vi "HAMEG_HMP2020.vi"() -> ()   [LabVIEW 2011, in "run.lvlib"]
uses:
  run.lvlib
panel:
  out "Boolean array":bool[](array[boolean])
  in  "Time":dbl[](array[numeric])=[0.1, 0.1]
  in  "Voltage":dbl[](array[numeric])=[0.5, 0.4] format="%.3f"
  in  "Current":dbl[](array[numeric])=[2.0, 2.0] format="%.3f"
  in  "Channel (Channel 1)":i32(ring)=1 items=["Channel 1"=1, "Channel 2"=2, "Channel 3"=3, "Channel 4"=4]
  in  "VISA resource name":refnum<visa-resource-name>="COM3"
  in  "stop":bool
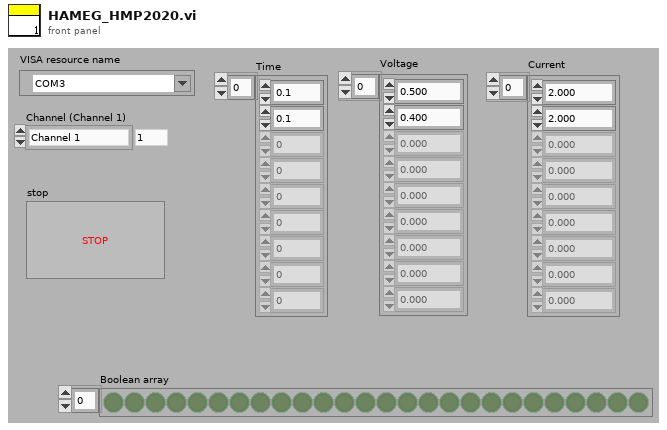
[diagram p1: front panel]
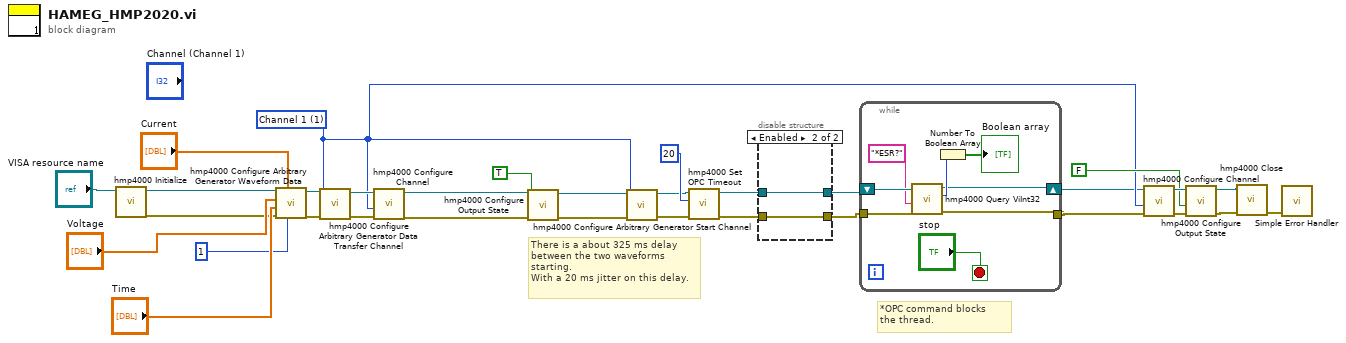
[diagram p0: block diagram]
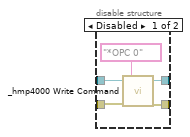
[diagram p2: hidden frame]
diagram:
  w3 = 1 items=["Channel 1"=1, "Channel 2"=2, "Channel 3"=3, "Channel 4"=4] ("Channel (Channel 1)")
  # "*OPC command blocks \nthe thread."
  # "There is a about 325 ms delay\nbetween the two waveforms \nstarting.\nWith a 20 ms jitter on this delay."
  n1 = call <instrlib>:"hmp4000 Initialize.vi"("VISA resource name"="VISA resource name") -> ("error out"=w4:errorcluster, "VISA resource name out"=w5:refnum<visa-resource-name>)  [unwired: 9 in]
  n2 = call <instrlib>:"hmp4000 Configure Arbitrary Generator Waveform Data.vi"("Repetition (0)"=1, "Current"="Current", "error in (no error)"=w4, "Time"="Time", "Voltage"="Voltage", "VISA resource name"=w5) -> ("error out"=w25:errorcluster, "VISA resource name out"=w26:refnum<visa-resource-name>)  [unwired: 4 in]
  n3 = call <instrlib>:"hmp4000 Configure Arbitrary Generator Data Transfer Channel.vi"("error in (no error)"=w25, "Channel (Channel 1)"=w3, "VISA resource name"=w26) -> ("error out"=w24:errorcluster, "VISA resource name out"=w23:refnum<visa-resource-name>)  [unwired: 7 in]
  n4 = call <instrlib>:"hmp4000 Configure Channel.vi"("error in (no error)"=w24, "Channel (Channel 1)"=w3, "VISA resource name"=w23) -> ("error out"=w6:errorcluster, "VISA resource name out"=w7:refnum<visa-resource-name>)  [unwired: 7 in]
  n5 = call <instrlib>:"hmp4000 Configure Output State.vi"("error in (no error)"=w6, "Output State (Off)"=TRUE, "VISA resource name"=w7) -> ("error out"=w8:errorcluster, "VISA resource name out"=w9:refnum<visa-resource-name>)  [unwired: 7 in]
  n6 = call <instrlib>:"hmp4000 Configure Arbitrary Generator Start Channel.vi"("error in (no error)"=w8, "Channel (Channel 1)"=w3, "VISA resource name"=w9) -> ("error out"=w16:errorcluster, "VISA resource name out"=w17:refnum<visa-resource-name>)  [unwired: 7 in]
  n7 = call <instrlib>:"hmp4000 Set OPC Timeout.vi"("error in (no error)"=w16, "OPC Timeout"=u32 20, "VISA resource name"=w17) -> ("error out"=w28:errorcluster, "VISA resource name out"=w29:refnum<visa-resource-name>)  [unwired: 7 in]
  n8 = disable-structure shown="Enabled" {
    disable-tunnel: [w33 w38] -> w15
    disable-tunnel: [w34 w39] -> w30
    disable-tunnel: w29 -> [w37 w39]
    disable-tunnel: w28 -> [w36 w38]
    frame Disabled {
      n9 = call <instrlib>:"_hmp4000 Write Command.vi"("error in (no error)"=w36, "Command"="*OPC 0", "VISA resource name"=w37) -> ("error out"=w33:errorcluster, "VISA resource name out"=w34:refnum<visa-resource-name>)  [unwired: 7 in]
    }
    frame Enabled {
    }
  }
  n10 = while {
    shift-right: [w41] -> w2
    shift-left: w30 -> [w46]
    tunnel: w15 -> [w45]
    tunnel: [w40] -> w1
    stop <- "stop" stop-if-true
    n11 = call <instrlib>:"hmp4000 Query ViInt32.vi"("error in (no error)"=w45, "Command (\"\")"="*ESR?", "VISA resource name"=w46) -> ("error out"=w40:errorcluster, "Value"=w42:i32, "VISA resource name out"=w41:refnum<visa-resource-name>)  [unwired: 6 in]
    n12 = Number To Boolean Array(number=w42) -> (Boolean array=→"Boolean array":bool[])
  }
  n13 = call <instrlib>:"hmp4000 Configure Channel.vi"("error in (no error)"=w1, "Channel (Channel 1)"=w3, "VISA resource name"=w2) -> ("error out"=w13:errorcluster, "VISA resource name out"=w14:refnum<visa-resource-name>)  [unwired: 7 in]
  n14 = call <instrlib>:"hmp4000 Configure Output State.vi"("error in (no error)"=w13, "Output State (Off)"=FALSE, "VISA resource name"=w14) -> ("error out"=w10:errorcluster, "VISA resource name out"=w11:refnum<visa-resource-name>)  [unwired: 7 in]
  n15 = call <instrlib>:"hmp4000 Close.vi"("error in (no error)"=w10, "VISA resource name"=w11) -> ("error out"=w31:errorcluster)  [unwired: 9 in]
  n16 = call <vilib>:"Simple Error Handler.vi"("error in (no error)"=w31) -> ()  [unwired: 4 in, 5 out]
